vi "复件 Clear-Receive.vi"(8 "错误输入（无错误）":errorcluster, 10 "CANChannel":u32, 11 "DeviceType":T1=3 items=["PCI-CAN200"=7, "USB-CAN"=2, "USB-CAN200"=3]) -> (0 "错误输出":errorcluster, 1 "VCI_CAN_OBJ_R":T3={"ID"=96, 0, 0, 0, "TimeStamp"=0, "TimeFlag"=0, "SendType"=0, "RemoteFlag"=0, "ExternFlag"=0, "DataLen"=8, "Byte0"=0, "Byte1"=248, "Byte2"=17, "Byte3"=0, "Byte4"=0, "Byte5"=0, "Byte6"=0, "Byte7"=0, "Channel"=0, 77, 32} {"Byte7" format="%x"; "Byte6" format="%x"; "Byte5" format="%x"; "Byte4" format="%x"; "Byte3" format="%x"; "Byte2" format="%x"; "Byte1" format="%x"; "Byte0" format="%x"}, 2 "Result":bool=TRUE, 3 "DeviceTypeOut":u16(ring)=7 items=["PCI-CAN200"=7], 5 "每次接收完时间":u32)   [LabVIEW 2013]
uses:
  DevType.ctl
  VCI_CAN.dll
panel:
  out "VCI_CAN_OBJ_R 2":T2(array[cluster])
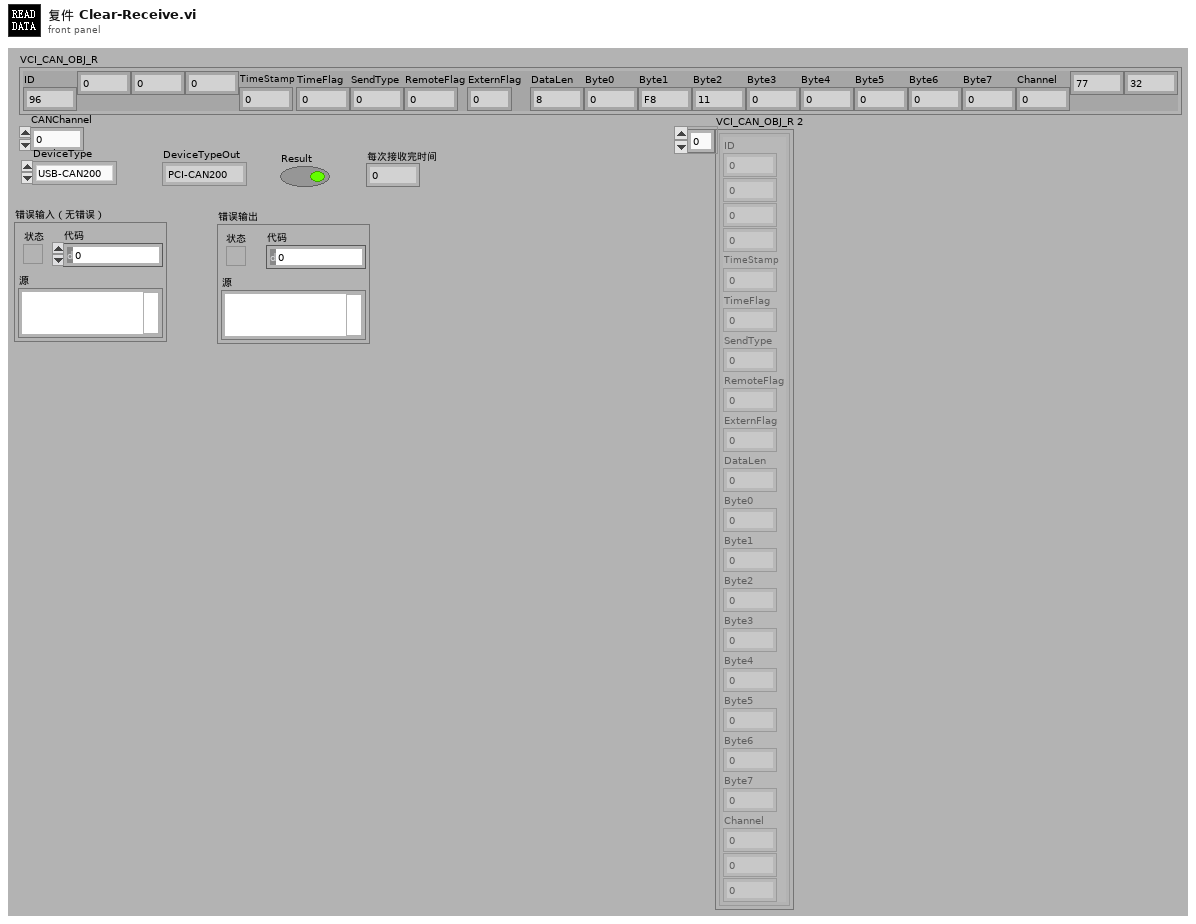
[diagram p1: front panel]
types:
  T1 = typedef "DevType.ctl" = u16
  T2 = cluster{"ID":u8, u8, u8, u8, "TimeStamp":u32, "TimeFlag":u8, "SendType":u8, "RemoteFlag":u8, "ExternFlag":u8, "DataLen":u8, "Byte0":u8, "Byte1":u8, "Byte2":u8, "Byte3":u8, "Byte4":u8, "Byte5":u8, "Byte6":u8, "Byte7":u8, "Channel":u8, u8, u8}[]
  T3 = cluster{"ID":u8, u8, u8, u8, "TimeStamp":u32, "TimeFlag":u8, "SendType":u8, "RemoteFlag":u8, "ExternFlag":u8, "DataLen":u8, "Byte0":u8, "Byte1":u8, "Byte2":u8, "Byte3":u8, "Byte4":u8, "Byte5":u8, "Byte6":u8, "Byte7":u8, "Channel":u8, u8, u8}
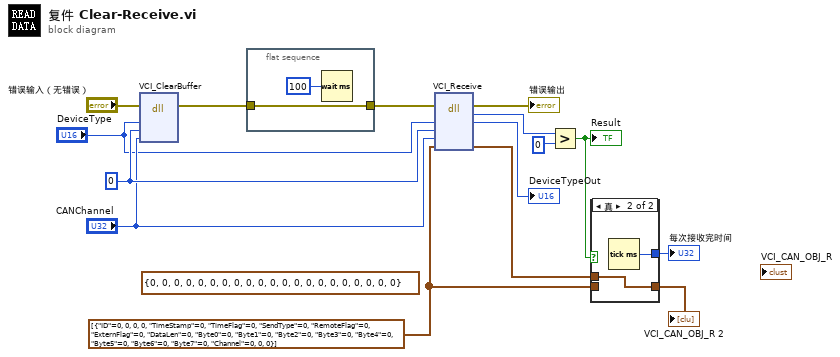
[diagram p0: block diagram]
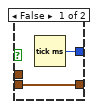
[diagram p2: hidden frame]
diagram:
  w3 = T2 [{"ID"=0, 0, 0, 0, "TimeStamp"=0, "TimeFlag"=0, "SendType"=0, "RemoteFlag"=0, "ExternFlag"=0, "DataLen"=0, "Byte0"=0, "Byte1"=0, "Byte2"=0, "Byte3"=0, "Byte4"=0, "Byte5"=0, "Byte6"=0, "Byte7"=0, "Channel"=0, 0, 0}]
  (unwired) T3 {"ID"=0, 0, 0, 0, "TimeStamp"=0, "TimeFlag"=0, "SendType"=0, "RemoteFlag"=0, "ExternFlag"=0, "DataLen"=0, "Byte0"=0, "Byte1"=0, "Byte2"=0, "Byte3"=0, "Byte4"=0, "Byte5"=0, "Byte6"=0, "Byte7"=0, "Channel"=0, 0, 0} ("VCI_CAN_OBJ_R 2")
  w10 = 0
  n1 = dll-call lib="PTH1Qabs D导航T-BOXT-BOX TestSystemInstrumentDriversUSB-CANVCI_CAN.dll" fn="VCI_ClearBuffer"(error in="错误输入（无错误）", "DeviceType"="DeviceType", "DeviceInd"=w10, "CANInd"="CANChannel") -> (error out=w9:errorcluster)  [unwired: 6 in, 1 out]
  n2 = flat-sequence {
    tunnel: w9 -> [w16]
    tunnel: [w16] -> w8
    frame #0 {
      n3 = Wait (ms)(milliseconds to wait=u32 100 ("等待时间（毫秒）")) -> ()  [unwired: 1 out]
    }
  }
  n4 = dll-call lib="PTH1Qabs D导航T-BOXT-BOX TestSystemInstrumentDriversUSB-CANVCI_CAN.dll" fn="VCI_Receive"(error in=w8, "DeviceType"="DeviceType", "DeviceInd"=w10, "CANInd"="CANChannel", "VCI_CAN_OBJ_R"=w3) -> (error out=→"错误输出":errorcluster, "返回类型"=w13:u32, "DeviceType"=→"DeviceTypeOut":u32, "VCI_CAN_OBJ_R"=w5:T2)  [unwired: 4 in, 1 out]
  n5 = Greater?(x=w13, y=u32 0) -> (0:w6:bool)
  "Result" <- w6
  n6 = case shown="真" w6 {
    tunnel: w5 -> [_ w21]
    tunnel: [w19 w21] -> w2
    tunnel: w3 -> [w19 _]
    tunnel: [w18 w20] -> w4
    frame False {
      n7 = Tick Count (ms)() -> (millisecond timer value=w18:u32)
    }
    frame True {
      n8 = Tick Count (ms)() -> (millisecond timer value=w20:u32)
    }
  }
  "每次接收完时间" <- w4
  "VCI_CAN_OBJ_R 2" <- w2
